vi "Rx Async.vi"(8 "error in (no error)":errorcluster, 10 "Dispatcher Interface in":refnum<class "Dispatcher Interface.lvclass">, 11 "Plugin in":refnum<class "Plugin.lvclass">) -> (0 "error out":errorcluster, 2 "Dispatcher Interface out":refnum<class "Dispatcher Interface.lvclass">, 3 "Plugin out":refnum<class "Plugin.lvclass">)   [LabVIEW 2017, in "DSF Core.lvlib" / "Plugin.lvclass"]
uses:
  Plugin.lvclass
  Interfaces/Dispatcher/Dispatcher Interface.lvclass
  C:/Git/DSF/Data Sharing Framework/Source/Core/Classes/Interfaces/Interface/Interface.lvclass
  Plugin.lvclass/Plugin.ctl
  Transfer Group/Transfer Group.lvclass/Transfer Group.ctl
  Timing/Timing.lvclass/Timing.ctl
  Interfaces/Dispatcher/Command.ctl
  Buffers/Buffers.lvclass/Buffers.ctl
  <vilib>/NI/Memory Manager/Classes/Pointer/Pointer.lvclass/Pointer.ctl
  Interfaces/Interface/Interface.lvclass/Interface.ctl
  Interfaces/Dispatcher/Send Dispatcher Command.vi
  Transfer Group/Retrieve from FIFO.vi
  Transfer Group Status/Write Status.vi
  <vilib>/NI/Memory Manager/Classes/Pointer/Copy All.vi
  Interfaces/Dispatcher/Write.vi
  Interfaces/Dispatcher/Write Dispatcher Command.vi
  Transfer Group/Read Return FIFO.vi
  Transfer Group/Increment Late Count.vi
  <vilib>/NI/Memory Manager/Classes/Pointer/Check Size (0D).vi
  <vilib>/NI/Memory Manager/Classes/Pointer/Get Address.vi
  Transfer Group Status/Status Size.vi
  <vilib>/NI/Memory Manager/Classes/Pointer/Get Size.vi
  <vilib>/NI/Memory Manager/Classes/Pointer/Copy.vi
  Interfaces/Interface/Send Command.vi
  <vilib>/NI/Memory Manager/Classes/Pointer/Errors.vi
  <vilib>/NI/Memory Manager/Classes/Pointer/Out of Bounds.vi
  <vilib>/NI/Memory Manager/Classes/Pointer/Copy (No Check).vi
  <vilib>/NI/Memory Manager/Classes/Pointer/Check Pointer Bounds.vi
  <vilib>/NI/Memory Manager/Classes/Pointer/Check Null Pointer.vi
  Interfaces/Interface/Write RT FIFO.vi
  <vilib>/NI/Memory Manager/VIs/Source.Write.String.vi
  <vilib>/NI/Memory Manager/Classes/Pointer/Write Pointer Size.vi
  <vilib>/NI/Memory Manager/Classes/Pointer/Create Error.vi
  <vilib>/NI/Memory Manager/VIs/Source.Write.Scalar.Base10.vi
  <vilib>/NI/Memory Manager/VIs/Source.Write.Scalar.Base10 (U64).vi
  <vilib>/NI/Memory Manager/Classes/Pointer/Null Pointer.vi
  <vilib>/NI/Memory Manager/Classes/Pointer/Is Null.vi
  <vilib>/NI/Memory Manager/VIs/New Error Cluster Constant.vi
  <vilib>/NI/Memory Manager/VIs/New Error Cluster Constant (512B).vi
  <vilib>/NI/Memory Manager/VIs/Error Cluster.Set Status.vi
  <vilib>/NI/Memory Manager/VIs/Error Cluster.Set Code.vi
  <vilib>/NI/Memory Manager/VIs/Error Cluster.Set VI Source.vi
  <vilib>/NI/Memory Manager/Constants/Constants.vi
  <vilib>/NI/Memory Manager/Constants/Library Name.vi
  <vilib>/NI/Memory Manager/Classes/Pointer/Pointer Error Info.vi
  <vilib>/NI/Memory Manager/Constants/Pointer Class Name.vi
  Buffer/Buffer.lvclass
  C:/Program Files (x86)/National Instruments/LabVIEW 2017/vi.lib/NI/Memory Manager/Classes/Pointer/Pointer.lvclass
  Transfer Group Status/Status.lvclass
  Interfaces/Interface/Errors.vi
  Interfaces/Dispatcher/Command Timeout.vi
  VIs/VI Name.vi
  Interfaces/Dispatcher/Class Name.vi
  Transfer Group/Errors.vi
  Transfer Group/Return Timeout Error.vi
  Transfer Group/Invalid Iteration Error.vi
  Transfer Group/Transfer Group.lvclass
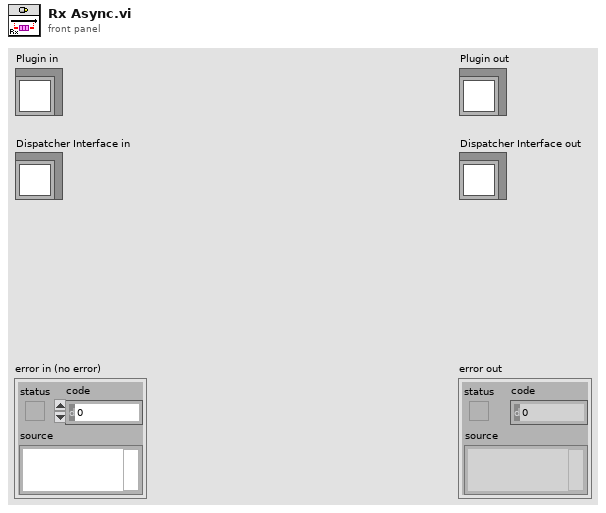
[diagram p1: front panel]
types:
  T1 = typedef "DSF Core.lvlib/Dispatcher Interface.lvclass/Command.ctl" = enum8{"Rx", "Tx", "Set Inline Buffer", "Shutdown"}
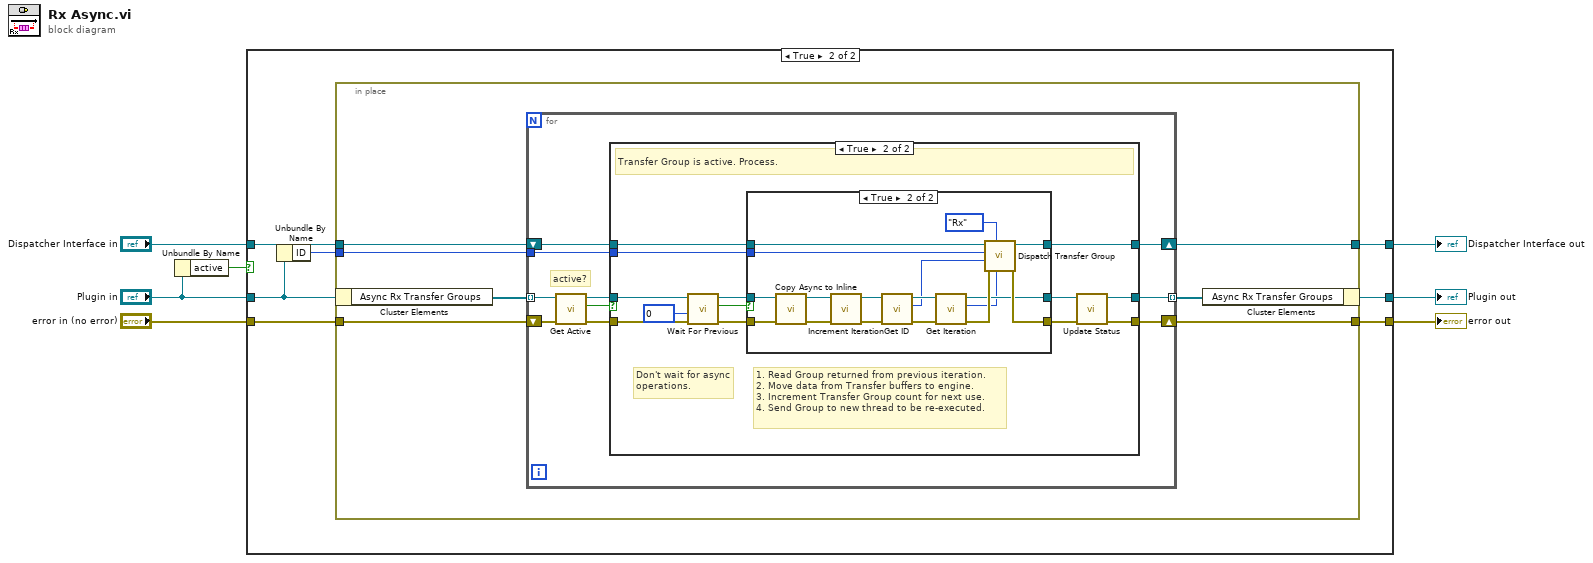
[diagram p0: block diagram]
diagram:
  n1 = Unbundle By Name("Plugin in") -> ("active"=w1:bool)
  n2 = case shown="True" w1 {
    tunnel: "error in (no error)" -> [w8 w17]
    tunnel: [w8 w16] -> w6
    tunnel: [w10 w15] -> w5
    tunnel: "Dispatcher Interface in" -> [w9 w14]
    tunnel: [w9 w13] -> w3
    tunnel: "Plugin in" -> [w10 w12]
    frame False {
    }
    frame True {
      n3 = Unbundle By Name(w12) -> ("ID"=w11:i32)
      n4 = in-place {
        in-place-border: w17 -> [w24]
        in-place-border: [w23] -> w16
        in-place-border: w14 -> [w20]
        in-place-border: [w19] -> w13
        in-place-border: w11 -> [w18]
        n5 = in-place-cluster #1(w12) -> ("Async Rx Transfer Groups"=w22:refnum<class "Transfer Group.lvclass">[])
        n6 = for {
          tunnel: w22 -> [w27] mode=indexing
          shift-right: [w33] -> w23
          shift-left: w24 -> [w32]
          tunnel: [w31] -> w21 mode=indexing
          shift-right: [w29] -> w19
          shift-left: w20 -> [w30]
          tunnel: w18 -> [w28]
          # "active?"
          n7 = call "Get Active.vi"("Transfer Group in"=w27) -> ("active"=w25:bool, "Transfer Group out"=w26:refnum<class "Transfer Group.lvclass">)  [unwired: 9 in]
          n8 = case shown="True" w25 {
            tunnel: [w36 w38] -> w33
            tunnel: w32 -> [w36 w48]
            tunnel: w26 -> [w35 w49]
            tunnel: [w35 w37] -> w31
            tunnel: w30 -> [w34 w43]
            tunnel: [w34 w44] -> w29
            tunnel: w28 -> [_ w42]
            frame False {
              # "Transfer Group is not active. Skip."
            }
            frame True {
              # "Don't wait for async operations."
              # "1. Read Group returned from previous iteration.\n2. Move data from Transfer buffers to engine.\n3. Increment Transfer Group count for next use.\n4. Send Group to new thread to be re-executed."
              # "Transfer Group is active. Process."
              n9 = call "Wait For Previous.vi"("error in (no error)"=w48, "timeout in ms (0)"=0, "Transfer Group in"=w49) -> ("error out"=w45:errorcluster, "ready"=w41:bool, "Transfer Group out"=w46:refnum<class "Transfer Group.lvclass">)  [unwired: 6 in]
              n10 = case shown="True" w41 {
                tunnel: w46 -> [w52 w68]
                tunnel: [w52 w57] -> w40
                tunnel: [w51 w58] -> w39
                tunnel: w45 -> [w51 w67]
                tunnel: [w50 w55] -> w44
                tunnel: w43 -> [w50 w54]
                tunnel: w42 -> [_ w53]
                frame False {
                }
                frame True {
                  n11 = call "Copy Async to Inline.vi"("error in (no error)"=w67, "Transfer Group in"=w68) -> ("error out"=w59:errorcluster, "Transfer Group out"=w60:refnum<class "Transfer Group.lvclass">)  [unwired: 8 in]
                  n12 = call "Increment Iteration.vi"("error in (no error)"=w59, "Transfer Group in"=w60) -> ("error out"=w64:errorcluster, "Transfer Group out"=w66:refnum<class "Transfer Group.lvclass">)  [unwired: 8 in]
                  n13 = call "Get ID.vi"("Transfer Group in"=w66) -> ("id"=w63:i32, "Transfer Group out"=w65:refnum<class "Transfer Group.lvclass">)  [unwired: 9 in]
                  n14 = call "Get Iteration.vi"("error in (no error)"=w64, "Transfer Group in"=w65) -> ("error out"=w62:errorcluster, "iteration"=w56:u64, "Transfer Group out"=w57:refnum<class "Transfer Group.lvclass">)  [unwired: 7 in]
                  n15 = call "Dispatch Transfer Group.vi"("Iteration"=w56, "command"=Command."Rx", "error in (no error)"=w62, "Transfer Group ID"=w63, "Plugin ID"=w53, "Dispatcher Interface in"=w54) -> ("error out"=w58:errorcluster, "Dispatcher Interface out"=w55:refnum<class "Dispatcher Interface.lvclass">)  [unwired: 4 in]
                }
              }
              n16 = call "Update Status.vi"("error in (no error)"=w39, "Transfer Group in"=w40) -> ("error out"=w38:errorcluster, "Transfer Group out"=w37:refnum<class "Transfer Group.lvclass">)  [unwired: 8 in]
            }
          }
        }
        n17 = in-place-cluster #1("Async Rx Transfer Groups"=w21) -> (w15:refnum<class "Plugin.lvclass">)
      }
    }
  }
  "error out" <- w6
  "Plugin out" <- w5
  "Dispatcher Interface out" <- w3
